vi "Update Dir Size.vi"(7 "Size":u32, 10 "Name":string, 11 "Map":T1) -> (3 "Map Out":T1)   [LabVIEW 2020]
uses:
  MAP_Structure.ctl
  Cluster_Item Data.ctl
  <vilib>/Utility/miscctls.llb/LVMapReplaceAction.ctl
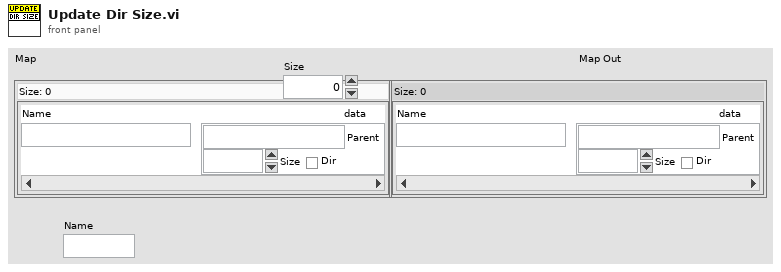
[diagram p1: front panel]
types:
  T1 = typedef "MAP_Structure.ctl" = map{string, T2}
  T2 = typedef "Cluster_Item Data.ctl" = cluster{"Parent":string, "Size":u32, "Dir":bool}
  T3 = typedef "LVMapReplaceAction.ctl" = enum32{"Modify Entry only if found", "Add or Modify Entry", "Delete Entry"}
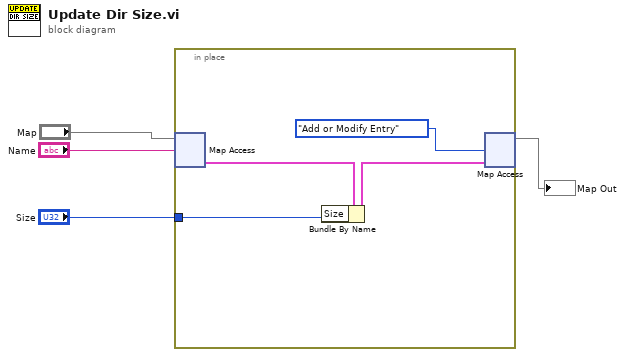
[diagram p0: block diagram]
diagram:
  n1 = in-place {
    in-place-border: "Size" -> [w5]
    n2 = in-place-map #1("Map", "Name") -> (w8:T2)  [unwired: 1 in, 1 out]
    n3 = Bundle By Name(cluster=w8, "Size"=w5) -> (w7:T2)
    n4 = in-place-map #1(w7, LVMapReplaceAction."Add or Modify Entry" ("action")) -> (→"Map Out":T1)  [unwired: 2 out]
  }
